vi "record shoulder.vi"(9 "Record":bool, 10 "EncoderDevRef":T1={"DevStatus"={"status"=FALSE, "code"=0, "source"=""}, "EncoderIndex"=enum."Enc 0", "CounterIndex"=enum."Invalid", "DistancePerCount"=1.0, "Decoding Type"=enum."4x"}) -> (1 "New Recording":bool, 2 "Encoder Recording Data":cluster{dbl, u32}[](array[cluster])=[{0.0, 104}, {0.0, 201}, {0.0, 301}, {0.0, 407}, {0.0, 507}, {0.0, 603}, {0.0, 705}, {0.0, 805}, {0.0, 909}, {0.0, 1006}, {0.0, 1104}, {0.0, 1205}, {0.0, 1312}, {0.0, 1408}, {0.0, 1511}, {0.0, 1608}, {0.0, 1715}, {0.0, 1810}, {0.0, 1910}, {0.0, 2011}, {-0.25, 2110}, {-0.25, 2210}, {-0.25, 2309}, {-0.25, 2411}, {-0.25, 2511}, {-4.0, 2613}, {-12.25, 2712}, {-12.25, 2811}, {83.5, 2912}, {419.5, 3014}, {761.0, 3112}, {1215.75, 3215}, {1565.5, 3315}, {1883.0, 3417}, {2263.0, 3517}, {2699.5, 3619}, {3125.75, 3717}, {3586.75, 3817}, {4020.0, 3917}, {4329.5, 4017}, {4659.0, 4118}, {5082.0, 4219}, {5512.25, 4318}, {5925.0, 4419}, {6361.5, 4524}, {6790.75, 4620}, {7260.75, 4720}, {7728.0, 4819}, {8201.75, 4919}, {8703.5, 5021}, {9211.75, 5124}, {9709.75, 5223}, {10202.0, 5321}, {10723.5, 5423}, {11231.5, 5520}, {11762.25, 5621}, {12321.25, 5725}, {12872.5, 5823}, {13459.0, 5927}, {14014.75, 6026}, {14574.25, 6124}, {15166.0, 6225}, {15751.25, 6327}, {16338.0, 6425}, {16978.0, 6529}, {17593.5, 6628}, {18249.75, 6732}, {18889.0, 6829}, {19558.0, 6929}, {20259.0, 7032}, {20952.25, 7131}, {21656.75, 7231}, {22384.0, 7331}, {23164.0, 7435}, {23908.5, 7534}, {24671.0, 7634}, {25446.25, 7735}, {26218.75, 7835}, {26986.25, 7934}, {27775.25, 8034}, {28573.0, 8135}, {29093.25, 8236}, {29439.5, 8335}, {29533.75, 8436}, {29578.75, 8537}, {29697.75, 8640}, {29835.0, 8740}, {30049.75, 8840}, {30444.5, 8943}, {30919.75, 9042}, {31488.0, 9142}, {32109.25, 9241}, {32794.25, 9343}, {33484.5, 9443}, {34199.75, 9544}, {34944.25, 9645}, {35705.0, 9744}, {36496.5, 9844}, {37365.75, 9948}, {38152.75, 10046}, {38947.0, 10145}, {39719.5, 10245}, {40546.25, 10352}, {41281.0, 10449}, {42031.0, 10547}, {42819.75, 10650}, {43258.75, 10749}, {43335.0, 10849}, {43335.25, 10949}, {43335.25, 11049}, {43335.25, 11148}, {43335.25, 11248}, {43335.25, 11350}, {43335.25, 11451}, {43335.25, 11554}, {43335.25, 11650}, {43335.25, 11750}, {43335.25, 11852}, {43335.25, 11951}, {43335.25, 12051}, {43335.25, 12153}, {43335.25, 12253}, {43335.25, 12352}, {43335.25, 12452}, {43335.25, 12553}, {43335.25, 12655}, {43335.25, 12754}])   [LabVIEW 2017]
uses:
  <vilib>/Rock Robotics/WPI/Encoder/WPI_EncoderDevRef.ctl
  <vilib>/Rock Robotics/SystemInterfaces/Encoder/FPGA_EncoderIdx.ctl
  <vilib>/Rock Robotics/SystemInterfaces/Counter/FPGA_CounterCtrSystemIndex.ctl
  <vilib>/Rock Robotics/WPI/Encoder/WPI_EncoderType.ctl
panel:
  out "Elapsed Time":u32=12754
  out "Recording Graph":cluster{"Distance":dbl, u32}[](graph)=[{"Distance"=0.0, 104}, {"Distance"=0.0, 201}, {"Distance"=0.0, 301}, {"Distance"=0.0, 407}, {"Distance"=0.0, 507}, {"Distance"=0.0, 603}, {"Distance"=0.0, 705}, {"Distance"=0.0, 805}, {"Distance"=0.0, 909}, {"Distance"=0.0, 1006}, {"Distance"=0.0, 1104}, {"Distance"=0.0, 1205}, {"Distance"=0.0, 1312}, {"Distance"=0.0, 1408}, {"Distance"=0.0, 1511}, {"Distance"=0.0, 1608}, {"Distance"=0.0, 1715}, {"Distance"=0.0, 1810}, {"Distance"=0.0, 1910}, {"Distance"=0.0, 2011}, {"Distance"=-0.25, 2110}, {"Distance"=-0.25, 2210}, {"Distance"=-0.25, 2309}, {"Distance"=-0.25, 2411}, {"Distance"=-0.25, 2511}, {"Distance"=-4.0, 2613}, {"Distance"=-12.25, 2712}, {"Distance"=-12.25, 2811}, {"Distance"=83.5, 2912}, {"Distance"=419.5, 3014}, {"Distance"=761.0, 3112}, {"Distance"=1215.75, 3215}, {"Distance"=1565.5, 3315}, {"Distance"=1883.0, 3417}, {"Distance"=2263.0, 3517}, {"Distance"=2699.5, 3619}, {"Distance"=3125.75, 3717}, {"Distance"=3586.75, 3817}, {"Distance"=4020.0, 3917}, {"Distance"=4329.5, 4017}, {"Distance"=4659.0, 4118}, {"Distance"=5082.0, 4219}, {"Distance"=5512.25, 4318}, {"Distance"=5925.0, 4419}, {"Distance"=6361.5, 4524}, {"Distance"=6790.75, 4620}, {"Distance"=7260.75, 4720}, {"Distance"=7728.0, 4819}, {"Distance"=8201.75, 4919}, {"Distance"=8703.5, 5021}, {"Distance"=9211.75, 5124}, {"Distance"=9709.75, 5223}, {"Distance"=10202.0, 5321}, {"Distance"=10723.5, 5423}, {"Distance"=11231.5, 5520}, {"Distance"=11762.25, 5621}, {"Distance"=12321.25, 5725}, {"Distance"=12872.5, 5823}, {"Distance"=13459.0, 5927}, {"Distance"=14014.75, 6026}, {"Distance"=14574.25, 6124}, {"Distance"=15166.0, 6225}, {"Distance"=15751.25, 6327}, {"Distance"=16338.0, 6425}, {"Distance"=16978.0, 6529}, {"Distance"=17593.5, 6628}, {"Distance"=18249.75, 6732}, {"Distance"=18889.0, 6829}, {"Distance"=19558.0, 6929}, {"Distance"=20259.0, 7032}, {"Distance"=20952.25, 7131}, {"Distance"=21656.75, 7231}, {"Distance"=22384.0, 7331}, {"Distance"=23164.0, 7435}, {"Distance"=23908.5, 7534}, {"Distance"=24671.0, 7634}, {"Distance"=25446.25, 7735}, {"Distance"=26218.75, 7835}, {"Distance"=26986.25, 7934}, {"Distance"=27775.25, 8034}, {"Distance"=28573.0, 8135}, {"Distance"=29093.25, 8236}, {"Distance"=29439.5, 8335}, {"Distance"=29533.75, 8436}, {"Distance"=29578.75, 8537}, {"Distance"=29697.75, 8640}, {"Distance"=29835.0, 8740}, {"Distance"=30049.75, 8840}, {"Distance"=30444.5, 8943}, {"Distance"=30919.75, 9042}, {"Distance"=31488.0, 9142}, {"Distance"=32109.25, 9241}, {"Distance"=32794.25, 9343}, {"Distance"=33484.5, 9443}, {"Distance"=34199.75, 9544}, {"Distance"=34944.25, 9645}, {"Distance"=35705.0, 9744}, {"Distance"=36496.5, 9844}, {"Distance"=37365.75, 9948}, {"Distance"=38152.75, 10046}, {"Distance"=38947.0, 10145}, {"Distance"=39719.5, 10245}, {"Distance"=40546.25, 10352}, {"Distance"=41281.0, 10449}, {"Distance"=42031.0, 10547}, {"Distance"=42819.75, 10650}, {"Distance"=43258.75, 10749}, {"Distance"=43335.0, 10849}, {"Distance"=43335.25, 10949}, {"Distance"=43335.25, 11049}, {"Distance"=43335.25, 11148}, {"Distance"=43335.25, 11248}, {"Distance"=43335.25, 11350}, {"Distance"=43335.25, 11451}, {"Distance"=43335.25, 11554}, {"Distance"=43335.25, 11650}, {"Distance"=43335.25, 11750}, {"Distance"=43335.25, 11852}, {"Distance"=43335.25, 11951}, {"Distance"=43335.25, 12051}, {"Distance"=43335.25, 12153}, {"Distance"=43335.25, 12253}, {"Distance"=43335.25, 12352}, {"Distance"=43335.25, 12452}, {"Distance"=43335.25, 12553}, {"Distance"=43335.25, 12655}, {"Distance"=43335.25, 12754}]
  out "Encoder Distance":dbl=43335.25
  # "Record is used to start/stop recording\n-Starting a new recording wipes out the old one"
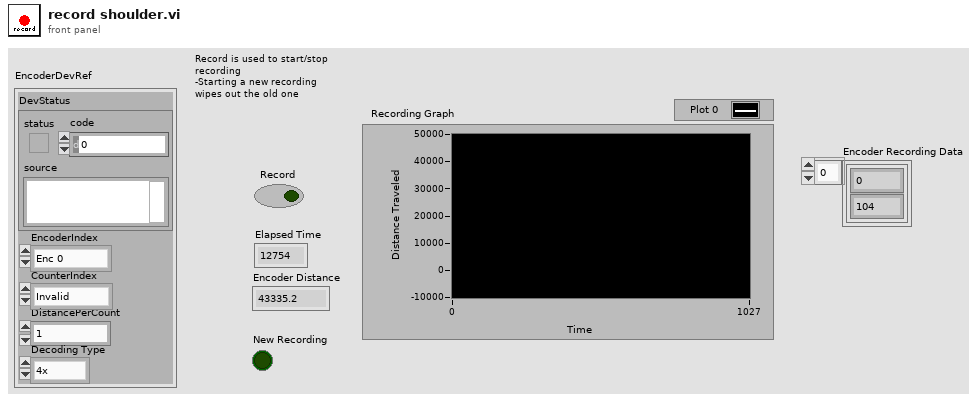
[diagram p1: front panel]
types:
  T1 = typedef "WPI_EncoderDevRef.ctl" = cluster{"DevStatus":errorcluster, "EncoderIndex":T2, "CounterIndex":T3, "DistancePerCount":dbl, "Decoding Type":T4}
  T2 = typedef "FPGA_EncoderIdx.ctl" = enum8{"Enc 0", "Enc 1", "Enc 2", "Enc 3", "Enc 4", "Enc 5", "Enc 6", "Enc 7", "Invalid"}
  T3 = typedef "FPGA_CounterCtrSystemIndex.ctl" = enum8{"Ctr 0", "Ctr 1", "Ctr 2", "Ctr 3", "Ctr 4", "Ctr 5", "Ctr 6", "Ctr 7", "Invalid"}
  T4 = typedef "WPI_EncoderType.ctl" = enum16{"1x", "2x", "4x"}
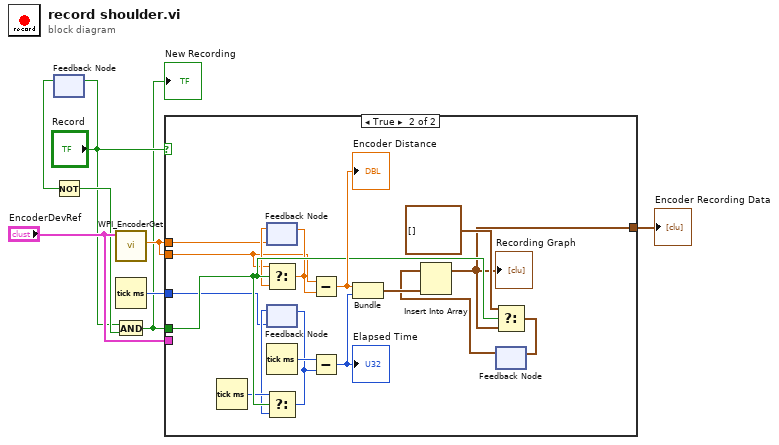
[diagram p0: block diagram]
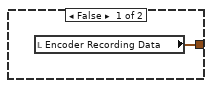
[diagram p2: hidden frame]
diagram:
  n1 = feedback-in #1("Record") -> ()
  n2 = feedback #1() -> (w4:bool)  [unwired: 1 in]
  n3 = Not(x=w4) -> (.not. x?=w3:bool)
  n4 = call <vilib>:"WPI_EncoderGet.vi"("EncoderDevRef"="EncoderDevRef") -> ("Distance"=w5:dbl)  [unwired: 5 in, 5 out]
  n5 = Tick Count (ms)() -> (millisecond timer value=w6:u32)
  n6 = And(x="Record", y=w3) -> (x .and. y?=w1:bool)
  "New Recording" <- w1
  n7 = case shown="True" "Record" {
    tunnel: "EncoderDevRef" -> [_ _]
    tunnel: [w9 w18] -> w7
    tunnel: w1 -> [_ w19]
    tunnel: w6 -> [_ w12]
    tunnel: w5 -> [_ w11]
    tunnel: w5 -> [_ w10]
    frame False {
      n8 = local read "Encoder Recording Data"() -> (w9:cluster{dbl, u32}[])
    }
    frame True {
      n9 = Tick Count (ms)() -> (millisecond timer value=w17:u32)
      n10 = feedback #2(w10) -> (w16:dbl)
      n11 = Select(t=w11, s=w19, f=w16) -> (s? t:f=w13:dbl)
      n12 = feedback-in #2(w13) -> ()
      n13 = feedback #3(w12) -> (w15:u32)
      n14 = Tick Count (ms)() -> (millisecond timer value=w25:u32)
      n15 = Select(t=w17, s=w19, f=w15) -> (s? t:f=w14:u32)
      n16 = feedback-in #3(w14) -> ()
      n17 = Subtract(x=w11, y=w13) -> (x-y=w23:dbl)
      "Encoder Distance" <- w23
      n18 = Subtract(x=w25, y=w14) -> (x-y=w24:u32)
      "Elapsed Time" <- w24
      n19 = Bundle(w23, w24) -> (w26:cluster{dbl, u32})  [unwired: 1 in]
      n20 = feedback #4() -> (w22:cluster{dbl, u32}[])  [unwired: 1 in]
      n21 = Insert Into Array(array=w22, new element=w26) -> (w18:cluster{dbl, u32}[])  [unwired: 1 in]
      "Recording Graph" <- w18
      n22 = Select(t=cluster{dbl, u32}[] [], s=w19, f=w18) -> (s? t:f=w20:cluster{dbl, u32}[])
      n23 = feedback-in #4(w20) -> ()
    }
  }
  "Encoder Recording Data" <- w7
